vi "Signal_acquisition_v3.vi"() -> ()   [LabVIEW 2015]
uses:
  <vilib>/measure/madcrms.llb/Basic Averaged DC-RMS for 1 Chan.vi
  <vilib>/measure/matone.llb/Extract Single Tone Information 1 Chan.vi
  <vilib>/express/express arith-compare/Formula/XNode/ExpressFormulaBlockNode.xnode
  <vilib>/measure/NI_MAPro.lvlib
panel:
  in  "Tab Control":T1(tab)
  in  "error in":errorcluster
  in  "Decimation":u16(ring)=8 items=["65536"=65535, "8192"=8192, "1024"=1024, "64"=64, "16"=8, "1"=1]
  in  "IP address":string="161.111.10.6"
  out "detected frequency":dbl format="%.2p"
  out "detected phase (deg)":dbl format="%.2p"
  in  "number \nof intervals":i32=60
  in  "FREQ START":i32=10000
  in  "FREQ END":i32=70000
  out "FRECUENCY END":i32
  in  "VOLTS ref":string="SOUR1:VOLT 0.1"
  in  "VOLTS":dbl=0.1
  out "error out":errorcluster
  in  "Pause \nfor buffer (ms) 2":u32=100
  in  "input 2":u16=1
  in  "Trigger Mode 2":string(combo)="CH1_NE"
  out "Voltage Gain / Frequency":cluster{i32, dbl}[](graph)
  out "Cutoff Freqs (Hz)":i32[](array[numeric])
  in  "MEASURE AMPLITUD":bool
  in  "SAVE DATA":bool
  out "Ieration\nnumber":i32
  out "millisecond \ntimer value":u32
  out "millisecond \nbegin timer":u32
  out "millisecond \nfinal timer":u32
  out "Acquisition\ntime complete":u32
  out "MEASURED amplitud":dbl format="%.2p"
  out "RESULT \nin amplittude":dbl
  in  "timeout ms":i32=2000
  in  "timeout ms\n (2000)":i32=2000
  in  "timeout ms\n (2000) 2":i32=2000
  in  "Delay\n (# Samples)":i32 max=16348
  in  "Trigger Level \n(0 mV)":i32
  out "REAL TIME MEASUREMENT":dbl[](graph)
  out "DC value 2":dbl format="%0.2p"
  out "detected \nfrequency 2":dbl format="%.2p"
  in  "FREQ START 5":i32
  in  "number of intervals  3":i32
  in  "number of intervals  2":i32
  # "FREQUENCY SWEEP"
  # "Settings parameters"
  # "FREQUENCY SWEEP"
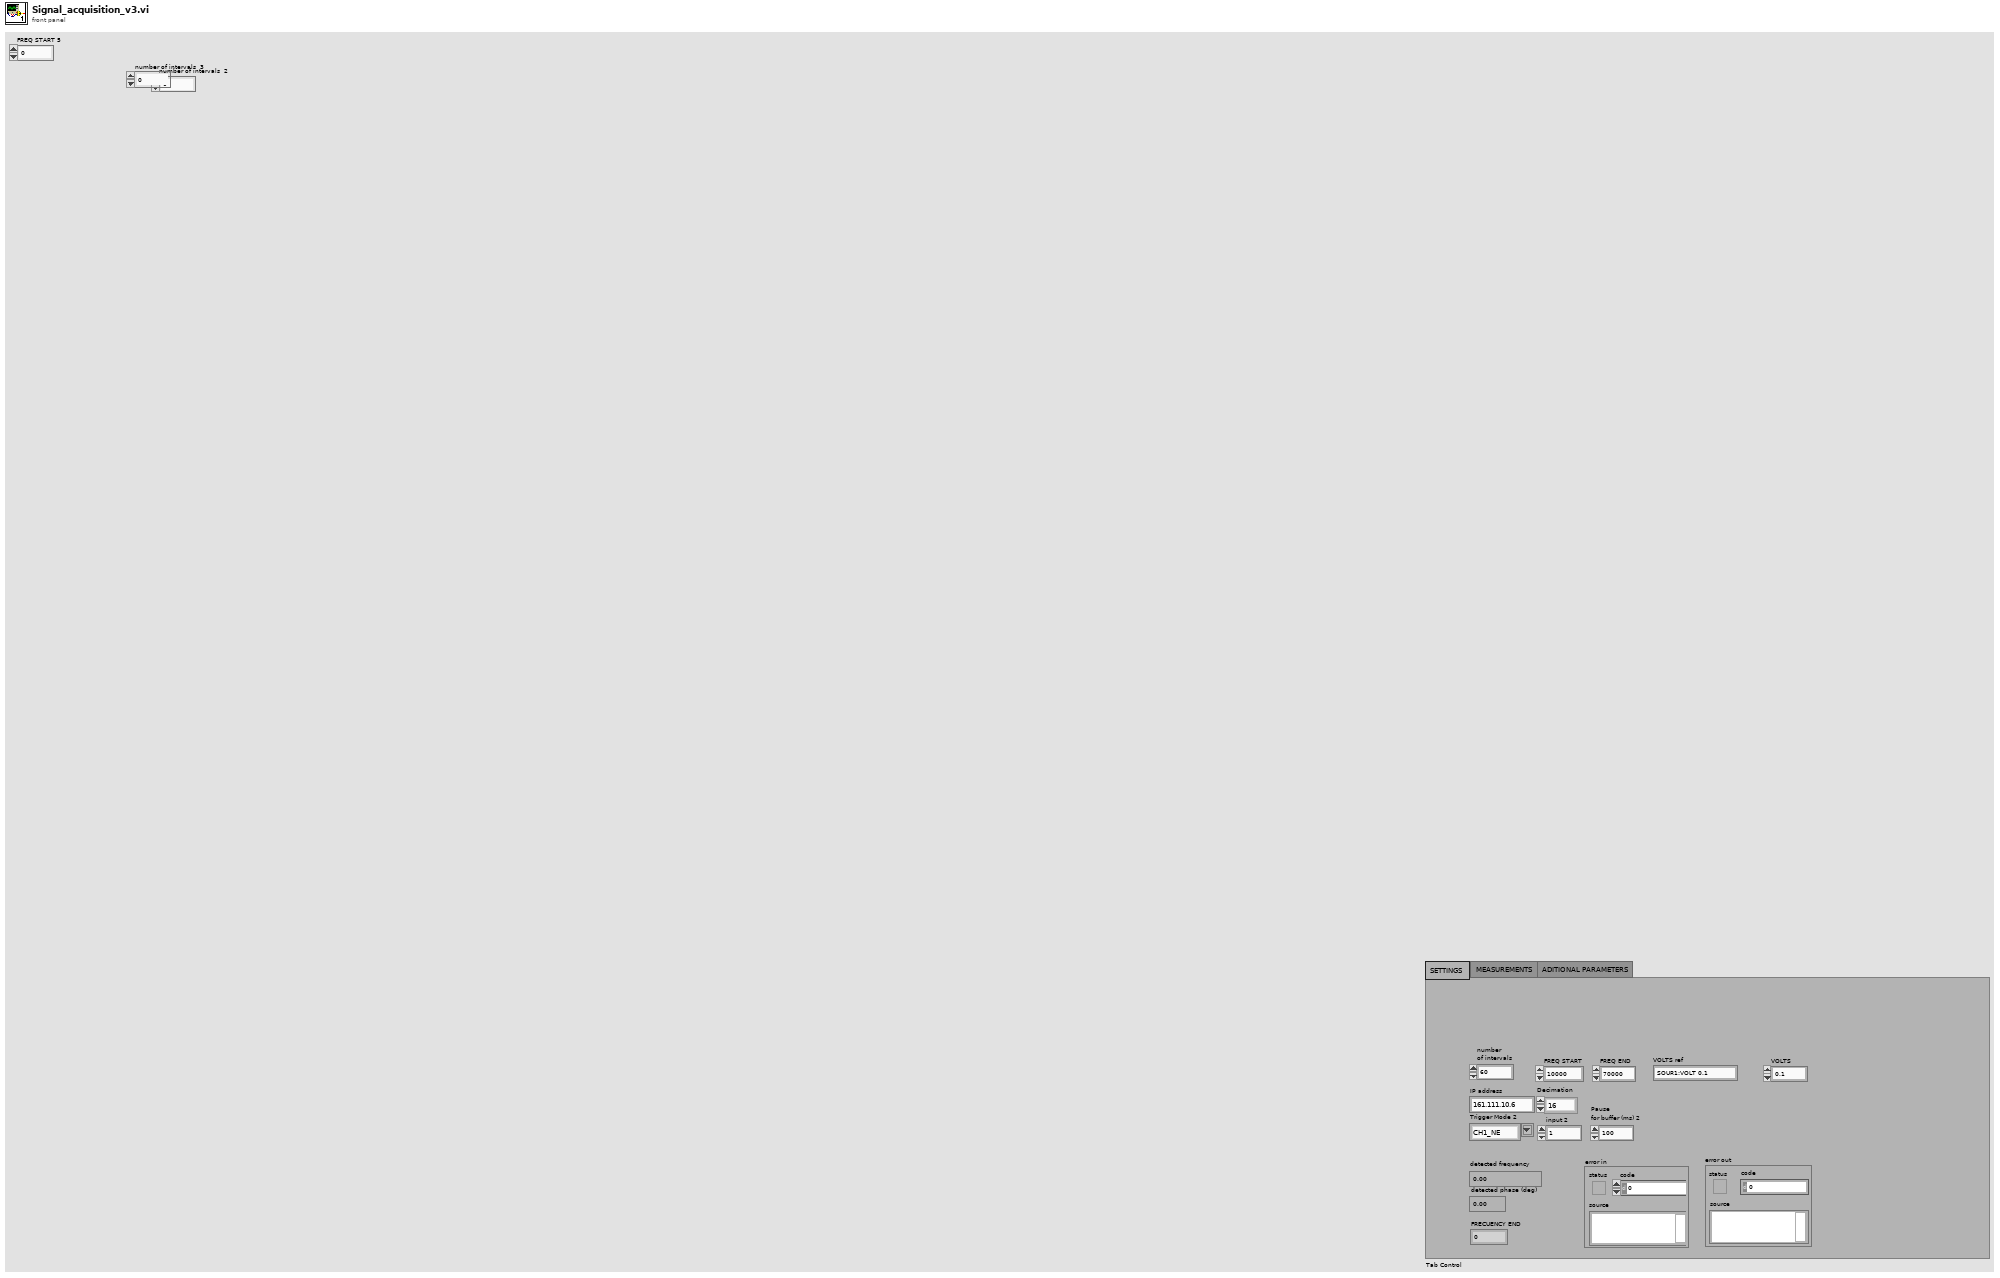
[diagram p1: front panel]
types:
  T1 = enum32{"SETTINGS ", "MEASUREMENTS ", "ADITIONAL PARAMETERS"}
  T2 = enum16{"Standard", "Buffered", "CRLF", "Immediate"}
  T3 = enum32{"none", "input signal", "detected signal", "residual signal"}
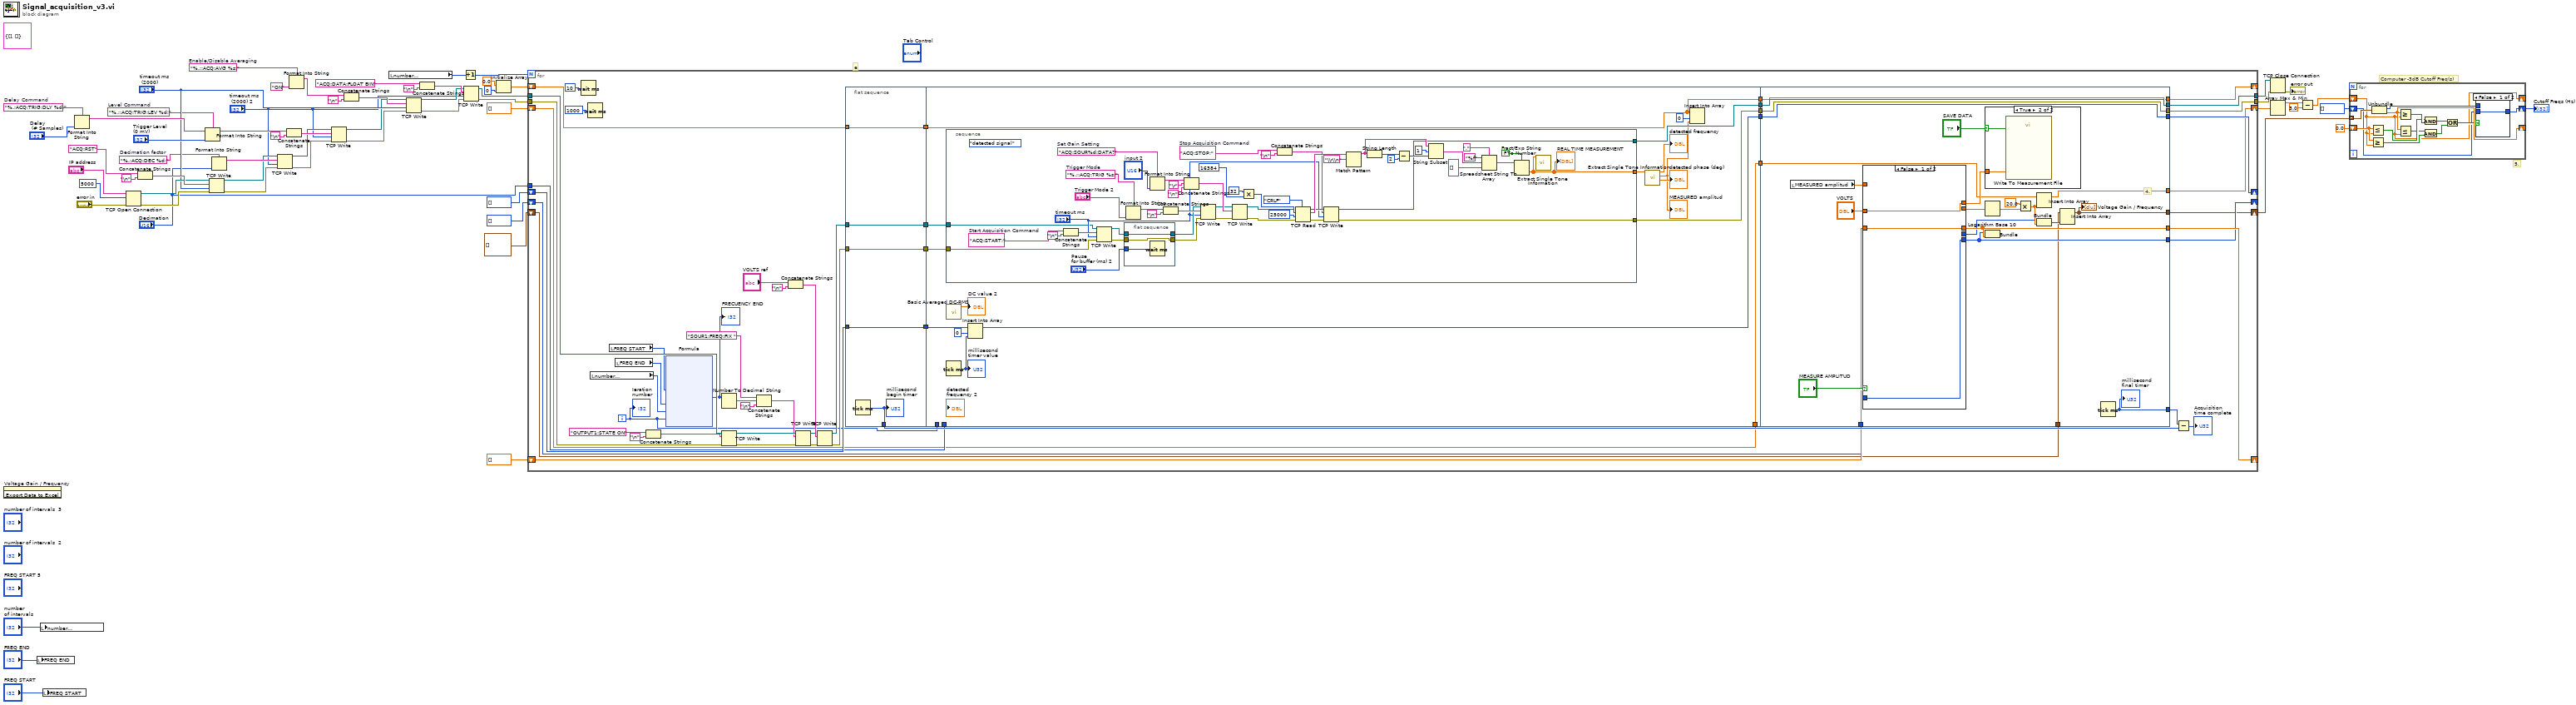
[diagram p0: block diagram]
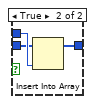
[diagram p2: hidden frame]
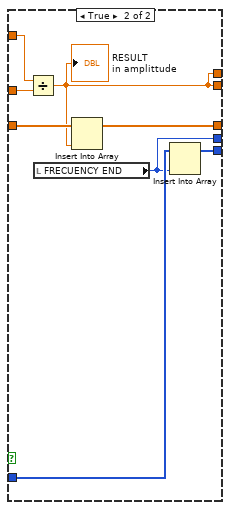
[diagram p4: hidden frame]
diagram:
  (unwired) cluster{dbl[], dbl[]} {[], []} ("FRECUENCY SWEEP")
  w29 = "%.;:ACQ:AVG %s;"  # Enable/Disable Averaging
  w37 = "%.;ACQ:DEC %d;"  # Decimation factor
  w38 = "%.;ACQ:TRIG:DLY %d;"  # Delay Command
  w39 = "%.;:ACQ:TRIG:LEV %d;"  # Level Command
  # "5."
  # "Computer -3dB Cutoff Freq(s)"
  # "e"
  n1 = invoke on="Voltage Gain / Frequency" class="XYGraph (strict)" method="Export Data to Excel"() -> ()  [unwired: 3 in, 3 out]
  n2 = local write "FREQ END"("FREQ END") -> ()
  n3 = local write "number \nof intervals"("number \nof intervals") -> ()
  n4 = local write "FREQ START"("FREQ START") -> ()
  n5 = Format Into String(format string=w38, "Delay\n (# Samples)") -> (resulting string=w57:string)  [unwired: 2 in, 1 out]
  n6 = TCP Open Connection(address="IP address", remote port or service name=u16 5000, error in (no error)="error in") -> (connection ID=w51:refnum<k5>, error out=w50:errorcluster)  [unwired: 2 in]
  n7 = Concatenate Strings("ACQ:RST" ("SCPI Message"), "\n") -> (w53:string)
  n8 = Format Into String(format string=w39, initial string=w57, "Trigger Level \n(0 mV)") -> (resulting string=w54:string)  [unwired: 1 in, 1 out]
  n9 = TCP Write(connection ID=w51, data in=w53, error in (no error)=w50, 9:"timeout ms\n (2000)") -> (connection ID out=w35:refnum<k5>, error out=w34:errorcluster)  [unwired: 1 out]
  n10 = Format Into String(format string=w37, "Decimation") -> (resulting string=w36:string)  [unwired: 2 in, 1 out]
  n11 = TCP Write(connection ID=w35, data in=w36, error in (no error)=w34, 9:"timeout ms\n (2000) 2") -> (connection ID out=w33:refnum<k5>, error out=w32:errorcluster)  [unwired: 1 out]
  n12 = Concatenate Strings(w54, "\n") -> (w48:string)
  n13 = Format Into String(format string=w29, "ON") -> (resulting string=w60:string)  [unwired: 2 in, 1 out]
  n14 = TCP Write(connection ID=w33, data in=w48, error in (no error)=w32, 9:"timeout ms\n (2000) 2") -> (connection ID out=w31:refnum<k5>, error out=w30:errorcluster)  [unwired: 1 out]
  n15 = Concatenate Strings(w60, "\n") -> (w49:string)
  n16 = local read "number \nof intervals"() -> (w15:i32)
  n17 = TCP Write(connection ID=w31, data in=w49, error in (no error)=w30, 9:"timeout ms\n (2000)") -> (connection ID out=w27:refnum<k5>, error out=w26:errorcluster)  [unwired: 1 out]
  n18 = Concatenate Strings("ACQ:DATA:FLOAT BIN" ("SCPI Message"), "\n") -> (w45:string)
  n19 = Increment(x=w15) -> (x+1=w14:i32)
  n20 = TCP Write(connection ID=w27, data in=w45, error in (no error)=w26, 9:"timeout ms\n (2000) 2") -> (connection ID out=w24:refnum<k5>, error out=w23:errorcluster)  [unwired: 1 out]
  n21 = Initialize Array(0.0 ("element"), 0 ("dimension size")) -> (w18:dbl[])
  n22 = for {
    N: w14 -> [_]
    tunnel: w24 -> [w86]
    tunnel: [w113] -> w44
    tunnel: [w112] -> w43
    tunnel: w23 -> [w83]
    shift-right: [w115] -> _
    shift-left: u32[] [] -> [w114]
    tunnel: "Decimation" -> [w102]
    shift-right: [w99] -> _
    shift-left: w18 -> [w97]
    shift-right: [w79] -> _
    shift-left: dbl[] [] -> [w80]
    shift-right: [w75] -> _
    shift-left: i32[] [] -> [w74]
    shift-right: [w69] -> w3
    shift-left: dbl[] [] -> [w67]
    shift-right: [w66] -> w2
    shift-left: cluster{"FRECUENCY END":i32, dbl}[] [] -> [w65]
    i -> [w73]
    n23 = Wait (ms)(milliseconds to wait=u32 10) -> ()  [unwired: 1 out]
    n24 = Wait (ms)(milliseconds to wait=u32 1000) -> ()  [unwired: 1 out]
    n25 = local read "number \nof intervals"() -> (w76:i32)
    n26 = local read "FREQ START"() -> (w77:i32)
    n27 = local read "FREQ END"() -> (w78:i32)
    n28 = Concatenate Strings("OUTPUT1:STATE ON" ("SCPI Message"), "\n") -> (w95:string)
    n29 = xnode "Formula"("Fin"=w77, "Fend"=w78, "Ninter"=w76, "i"=w73) -> ("Result"=w70:i32)  [unwired: 1 in, 1 out]
    "FRECUENCY END" <- w70
    n30 = Number To Decimal String(number=w70) -> (decimal integer string=w81:string)  [unwired: 1 in]
    n31 = TCP Write(connection ID=w86, data in=w95, error in (no error)=w83) -> (connection ID out=w92:refnum<k5>, error out=w91:errorcluster)  [unwired: 1 in, 1 out]
    n32 = Concatenate Strings("SOUR1:FREQ:FIX " ("SCPI Message"), w81, "\n") -> (w88:string)
    n33 = Concatenate Strings("VOLTS ref", "\n") -> (w87:string)
    n34 = TCP Write(connection ID=w92, data in=w88, error in (no error)=w91) -> (connection ID out=w72:refnum<k5>, error out=w71:errorcluster)  [unwired: 1 in, 1 out]
    n35 = TCP Write(connection ID=w72, data in=w87, error in (no error)=w71) -> (connection ID out=w85:refnum<k5>, error out=w84:errorcluster)  [unwired: 1 in, 1 out]
    n36 = flat-sequence {
      tunnel: w114 -> [w132]
      tunnel: w84 -> [w133]
      tunnel: w85 -> [w134]
      tunnel: [w134] -> w108
      tunnel: [w133] -> w107
      tunnel: [w132] -> w106
      tunnel: [w131] -> w104
      tunnel: [w130] -> w98
      tunnel: w97 -> [w130]
      tunnel: [w146] -> w111
      tunnel: [w144] -> w110
      tunnel: [w143] -> w109
      tunnel: w108 -> [w150]
      tunnel: w107 -> [w149]
      tunnel: w106 -> [w145]
      tunnel: w102 -> [_]
      tunnel: [w139] -> w100
      tunnel: w73 -> [_]
      tunnel: w98 -> [w139]
      tunnel: w67 -> [w135]
      tunnel: [w135] -> w68
      tunnel: [w227] -> w112
      tunnel: [w228] -> w113
      tunnel: [w229] -> w115
      tunnel: w111 -> [w229]
      tunnel: w110 -> [w228]
      tunnel: w109 -> [w227]
      tunnel: [w226] -> w105
      tunnel: w100 -> [w225]
      tunnel: [w225] -> w99
      tunnel: w80 -> [w220]
      tunnel: [w218] -> w79
      tunnel: [w217] -> w75
      tunnel: w74 -> [w219]
      tunnel: [w212] -> w69
      tunnel: w68 -> [w211]
      tunnel: [w209] -> w66
      tunnel: w65 -> [w208]
      frame #0 {
        n37 = Tick Count (ms)() -> (millisecond timer value=w131:u32)
        "millisecond \nbegin timer" <- w131
      }
      frame #1 {
        n38 = stacked-sequence {
          tunnel: w150 -> [w152]
          tunnel: w149 -> [w155]
          tunnel: [w153] -> w144
          tunnel: [w154] -> w143
          tunnel: [w151] -> w137
          frame #0 {
            w162 = "ACQ:STOP;"  # Stop Acquisition Command
            (unwired) T3."detected signal" ("export mode")
            w172 = "ACQ:SOUR%d:DATA?"  # Set Gain Setting
            w199 = "%.;:ACQ:TRIG %s;"  # Trigger Mode
            w201 = "ACQ:START;"  # Start Acquisition Command
            n39 = Concatenate Strings(w201, "\n") -> (w202:string)
            n40 = TCP Write(connection ID=w152, data in=w202, error in (no error)=w155, 9:"timeout ms") -> (connection ID out=w176:refnum<k5>, error out=w175:errorcluster)  [unwired: 1 out]
            n41 = flat-sequence {
              tunnel: "Pause \nfor buffer (ms) 2" -> [w205]
              tunnel: [w204] -> w174
              tunnel: [w203] -> w173
              tunnel: w176 -> [w204]
              tunnel: w175 -> [w203]
              frame #0 {
                n42 = Wait (ms)(milliseconds to wait=w205) -> ()  [unwired: 1 out]
              }
            }
            n43 = Format Into String(format string=w199, "Trigger Mode 2") -> (resulting string=w196:string)  [unwired: 2 in, 1 out]
            n44 = Format Into String(format string=w172, "input 2") -> (resulting string=w170:string)  [unwired: 2 in, 1 out]
            n45 = Concatenate Strings(w196, "\n") -> (w197:string)
            n46 = Concatenate Strings(w170, "\r", "\n") -> (w169:string)
            n47 = TCP Write(connection ID=w174, data in=w197, error in (no error)=w173, 9:"timeout ms") -> (connection ID out=w167:refnum<k5>, error out=w166:errorcluster)  [unwired: 1 out]
            n48 = TCP Write(connection ID=w167, data in=w169, error in (no error)=w166) -> (connection ID out=w168:refnum<k5>, error out=w165:errorcluster)  [unwired: 1 in, 1 out]
            n49 = Multiply(x=32, y=16384 ("bytes to read")) -> (x*y=w177:i32)
            n50 = Concatenate Strings(w162, "\n") -> (w160:string)
            n51 = TCP Read(connection ID=w168, bytes to read=w177, error in (no error)=w165, 7:T2."CRLF" ("mode (standard)"), 9:25000 ("timeout ms (25000)")) -> (connection ID out=w163:refnum<k5>, data out=w178:string, error out=w159:errorcluster)
            n52 = TCP Write(connection ID=w163, data in=w160, error in (no error)=w159, 9:"timeout ms") -> (connection ID out=w153:refnum<k5>, error out=w154:errorcluster)  [unwired: 1 out]
            n53 = Match Pattern(string=w178, regular expression="\\r\\n") -> (before substring=w184:string)  [unwired: 1 in, 3 out]
            n54 = String Length(string=w184) -> (length=w187:i32)
            n55 = Subtract(x=w187, y=2) -> (x-y=w188:i32)
            n56 = String Subset(string=w184, offset (0)=1, length (rest)=w188) -> (substring=w185:string)
            n57 = Spreadsheet String To Array(delimiter (Tab)=",", format string="%f", spreadsheet string=w185, array type (2D Dbl)=string[] [] ("Array")) -> (array=w191:string[])
            n58 = Fract/Exp String To Number(use system decimal point (T)=FALSE, string=w191) -> (number=w151:dbl[])  [unwired: 3 out]
            "REAL TIME MEASUREMENT" <- w151
            n59 = call-poly <vilib>:"Extract Single Tone Information.vi"("time signal in"=w151) -> ()  [unwired: 5 in, 6 out]
          }
        }
        n60 = call-poly <vilib>:"Basic Averaged DC-RMS.vi"() -> ("DC value"=→"DC value 2":dbl)  [unwired: 8 in, 3 out]
        n61 = Tick Count (ms)() -> (millisecond timer value=w147:u32)
        "millisecond \ntimer value" <- w147
        n62 = Insert Into Array(array=w145, index=0, new element=w147) -> (w146:u32[])
        n63 = call-poly <vilib>:"Extract Single Tone Information.vi"("time signal in"=w137) -> ("detected phase (deg)"=→"detected phase (deg)":dbl, "detected amplitude"=w136:dbl, "detected frequency"=→"detected frequency":dbl)  [unwired: 5 in, 3 out]
        "MEASURED amplitud" <- w136
        n64 = Insert Into Array(array=w139, index=0, new element=w136) -> ()  [unwired: 1 out]
      }
      frame #2 {
        # "4."
        n65 = local read "MEASURED amplitud"() -> (w224:dbl)
        n66 = case shown="False" "MEASURE AMPLITUD" {
          tunnel: w224 -> [_ w238]
          tunnel: [w232 w237] -> w222
          tunnel: w220 -> [w234 w242]
          tunnel: [w234 w241] -> w218
          tunnel: [w233 w240] -> w217
          tunnel: w219 -> [w233 w239]
          tunnel: [_ w237] -> w206
          tunnel: [_ w236] -> w210
          tunnel: "VOLTS" -> [w232 w235]
          frame False {
          }
          frame True {
            n67 = Divide(x=w238, y=w235) -> (x/y=w237:dbl)
            "RESULT \nin amplittude" <- w237
            n68 = local read "FRECUENCY END"() -> (w236:i32)
            n69 = Insert Into Array(array=w242, new element=w237) -> (w241:dbl[])  [unwired: 1 in]
            n70 = Insert Into Array(array=w239, new element=w236) -> (w240:i32[])  [unwired: 1 in]
          }
        }
        n71 = case shown="True" "SAVE DATA" {
          selector: "SAVE DATA" -> [_ w230]
          tunnel: w222 -> [_ w231]
          frame False {
          }
          frame True {
            n72 = call "Write To Measurement File"("Signals"=w231, "Enable"=w230) -> ()  [unwired: 15 in, 3 out]
          }
        }
        n73 = Logarithm Base 10(1:w206) -> (0:w214:dbl)
        n74 = Bundle(w217, w218) -> ()  [unwired: 1 in, 1 out]
        n75 = Multiply(x=20.0, y=w214) -> (x*y=w213:dbl)
        n76 = Insert Into Array(array=w211, new element=w213) -> (w212:dbl[])  [unwired: 1 in]
        n77 = Bundle("FRECUENCY END"=w210, w213) -> (w216:cluster{"FRECUENCY END":i32, dbl})  [unwired: 1 in]
        n78 = Insert Into Array(array=w208, new element=w216) -> (w209:cluster{"FRECUENCY END":i32, dbl}[])  [unwired: 1 in]
        "Voltage Gain / Frequency" <- w209
        n79 = Tick Count (ms)() -> (millisecond timer value=w226:u32)
        "millisecond \nfinal timer" <- w226
      }
    }
    n80 = Subtract(x=w105, y=w104) -> (x-y=→"Acquisition\ntime complete":u32)
    "Ieration\nnumber" <- w73
  }
  n81 = TCP Close Connection(connection ID=w44, error in (no error)=w43) -> (error out=→"error out":errorcluster)  [unwired: 1 in, 1 out]
  n82 = Array Max & Min(array=w3) -> (max value=w4:dbl)  [unwired: 3 out]
  n83 = Subtract(x=w4, y=3.0) -> (x-y=w5:dbl)
  n84 = for {
    tunnel: w2 -> [w256] mode=indexing
    shift-right: [w250] -> _
    shift-left: 0.0 -> [w251]
    shift-right: [w244] -> w7
    shift-left: i32[] [] -> [w245]
    shift-right: [w243] -> _
    shift-left: w5 -> [w243]
    n85 = Less Or Equal?(x=w251, y=w243) -> (x <= y?=w254:bool)
    n86 = Greater Or Equal?(x=w251, y=w243) -> (x >= y?=w252:bool)
    n87 = Unbundle(w256) -> ("FRECUENCY END"=w246:i32, w250:dbl)
    n88 = Greater Or Equal?(x=w250, y=w243) -> (x >= y?=w255:bool)
    n89 = Less Or Equal?(x=w250, y=w243) -> (x <= y?=w253:bool)
    n90 = And(x=w254, y=w255) -> (x .and. y?=w248:bool)
    n91 = And(x=w253, y=w252) -> (x .and. y?=w249:bool)
    n92 = Or(x=w248, y=w249) -> (x .or. y?=w247:bool)
    n93 = case shown="False" w247 {
      tunnel: w246 -> [_ w260]
      tunnel: w245 -> [w257 w259]
      tunnel: [w257 w258] -> w244
      frame False {
      }
      frame True {
        n94 = Insert Into Array(array=w259, new element=w260) -> (w258:i32[])  [unwired: 1 in]
      }
    }
  }
  "Cutoff Freqs (Hz)" <- w7
